vi "folder for output files.vi"(2 "results folder":path, 3 "folder name":string) -> (0 "appended path":path, 1 "Plug_in folder depth":i32)   [LabVIEW 2018]
uses:
  Globals/Plug_in_data_global.vi
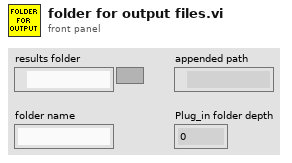
[diagram p1: front panel]
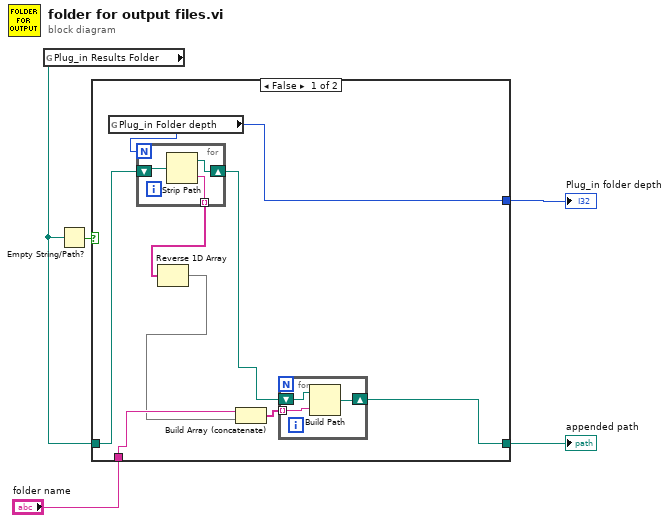
[diagram p0: block diagram]
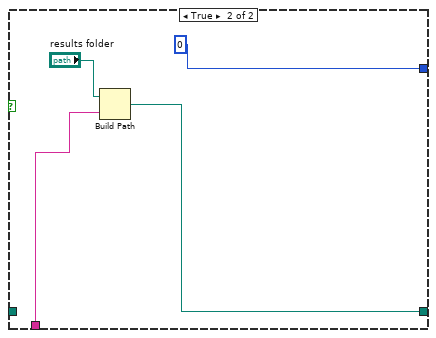
[diagram p2: hidden frame]
diagram:
  n1 = global read "Plug_in_data_global.vi" "Plug_in Results Folder"() -> (w2:path)
  n2 = Empty String/Path?(string/path=w2) -> (empty?=w1:bool)
  n3 = case shown="False" w1 {
    tunnel: [w10 w21] -> w5
    tunnel: w2 -> [w12 _]
    tunnel: [w13 0 ("Plug_in Folder depth")] -> w3
    tunnel: "folder name" -> [w9 w22]
    frame False {
      n4 = global read "Plug_in_data_global.vi" "Plug_in Folder depth"() -> (w13:i32)
      n5 = for {
        N: w13 -> [_]
        shift-right: [w18] -> w11
        shift-left: w12 -> [w19]
        tunnel: [w17] -> w7 mode=indexing
        n6 = Strip Path(path=w19) -> (stripped path=w18:path, name=w17:string)
      }
      n7 = Reverse 1D Array(array=w7) -> (reversed array=w6:string[])
      n8 = Build Array (concatenate)(w9, w6) -> (w8:string[])
      n9 = for {
        shift-right: [w14] -> w10
        shift-left: w11 -> [w16]
        tunnel: w8 -> [w15] mode=indexing
        n10 = Build Path(base path=w16, name or relative path=w15) -> (appended path=w14:path)
      }
    }
    frame True {
      n11 = Build Path(base path="results folder", name or relative path=w22) -> (appended path=w21:path)
    }
  }
  "appended path" <- w5
  "Plug_in folder depth" <- w3
